vi "Auto Gyro.vi"(8 "zeroGyro":dbl, 9 "headingTarget":dbl, 10 "xSpeed":dbl) -> (1 "Finished?":bool)   [LabVIEW 2016]
uses:
  Robot Global Data.vi
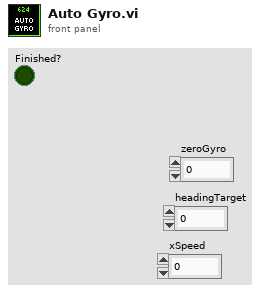
[diagram p1: front panel]
types:
  T1 = typedef "Dashboard Display Data.ctl" = cluster{"Climb Status Cluster":T2, "Drivetrain Status Cluster":T3, "Intake Status Cluster":T4, "Shooter Status Cluster":T8, "Drivetrain Encoder Values":T13, "Auton Command Cluster":T15, "Auton File Lists":T16}
  T2 = typedef "Climb Status Cluster.ctl" = cluster{"Climb Speed":dbl}
  T3 = typedef "Drivetrain Status Cluster.ctl" = cluster{"Drivetrain Mode":enum16{"Manual", "Gyro Steer"}, "Y (Throttle)":dbl, "X (Steer)":dbl, "Z (Strafe)":dbl, "Heading Target":dbl, "Center Piston Down?":bool, "Traction?":bool, "Gyro Steer Finished?":bool, "Distance Drive Finished?":bool, "Gyro":dbl, "Distance Target":dbl, "Y Max Output":dbl, "Y Min Output":dbl, "X Max Output":dbl, "X Min Output":dbl, "Z Max Output":dbl, "Z Min Output":dbl, "Translation Target":dbl, "Translation Drive Finished?":bool, "PID Auto Drive Finished?":bool, "Brake?":bool, "Vision Aligned?":bool}
  T4 = typedef "Intake Status Cluster.ctl" = cluster{"Roller Power":dbl, "Intake Mode":T5, "Intake Auto State":T6, "Backward Tripped?":bool, "Forward Tripped?":bool, "Filling Hopper?":bool, "Intake Current Trip State":T7, "Getting Gear?":bool, "Gear Slot Open":bool, "Wings Open":bool}
  T5 = typedef "Intake Modes.ctl" = enum16{"Manual", "Auto"}
  T6 = typedef "Intake Auto States.ctl" = enum16{"Outake Ball", "Idle", "Load Ball"}
  T7 = typedef "Intake Trip States.ctl" = enum16{"Normal", "Backward Tripped", "Forward Tripped"}
  T8 = typedef "Shooter Status Cluster.ctl" = cluster{"RPM":dbl, "Shooter RPM Ready?":bool, "Hopper Speed":dbl, "Shooter Mode":T9, "Shot Type":T10, "Shooter State":T11, "Motor Operational Status":T12}
  T9 = typedef "Shooter Modes.ctl" = enum16{"Auto", "Manual"}
  T10 = typedef "Shot Type.ctl" = enum16{"Dist Shot", "Key Shot"}
  T11 = typedef "Shooter Commands.ctl" = enum16{"Idle ", "Warmup ", "Shoot"}
  T12 = typedef "Shooter Motor Operational Status .ctl" = cluster{"Sensor Velocity ":dbl, "Encoder Position":dbl, "Encoder Velocity ":dbl, "Encoder Index Count":dbl, "Analog In":dbl, "Analog In Velocity":dbl, "Temperature (C)":dbl, "Temperature (K)":dbl, "Battery Voltage":dbl, "Current":dbl, "Sensor Position":dbl, "Vel Div 4":bool, "Encoder A Pin State":bool, "Encoder B Pin State":bool, "Encoder Index Pin State":bool, "Pulse Width Velocity ":dbl}
  T13 = typedef "Drivetrain Encoder Values.ctl" = cluster{"Left Encoder":T14, "Center Encoder":T14, "Right Encoder":T14}
  T14 = typedef "Encoder Values.ctl" = cluster{"Distance":dbl, "Speed":dbl, "Tick":dbl}
  T15 = typedef "Auton Command Cluster.ctl" = cluster{"commandID":dbl, "maxTime":dbl, "distanceTarget":dbl, "headingTarget":dbl, "translationTarget":dbl, "ySpeed":dbl, "xSpeed":dbl, "zSpeed":dbl, "async":dbl, "RPM":dbl, "Hood?":dbl, "Hopper?":dbl, "rollerPower":dbl, "fillHopper?":dbl, "zeroGyro":dbl}
  T16 = typedef "Auton File Lists.ctl" = cluster{"Current Queue":string, "General Scripts":string, "Movements":string}
  T17 = typedef "Drivetrain Command Cluster.ctl" = cluster{"Drivetrain Mode":T18, "Heading Target":dbl, "Turn Power":dbl, "Y Power":dbl, "Center Piston Down?":bool, "Traction?":bool, "Strafe Power":dbl, "Zero Gyro":bool, "Distance Target":dbl, "Strafe Correct":bool, "Y Max Output":dbl, "Y Min Output":dbl, "X Max Output":dbl, "X Min Output":dbl, "Z Max Output":dbl, "Z Min Output":dbl, "Z Target":dbl, "Brake?":bool}
  T18 = typedef "Drivetrain Mode.ctl" = enum16{"Manual", "Gyro Steer", "Distance Drive", "Translate Drive", "Goal Vision Align", "PID Drive"}
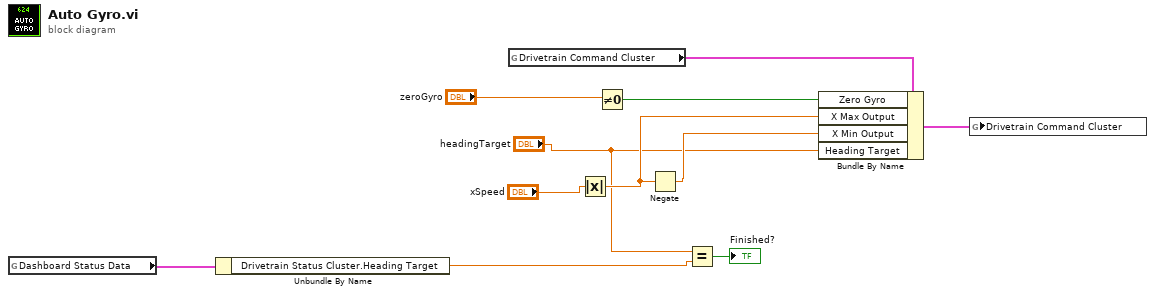
[diagram p0: block diagram]
diagram:
  n1 = global read "Robot Global Data.vi" "Dashboard Status Data"() -> (w9:T1)
  n2 = Unbundle By Name(w9) -> ("Drivetrain Status Cluster.Heading Target"=w3:dbl)
  n3 = global read "Robot Global Data.vi" "Drivetrain Command Cluster"() -> (w11:T17)
  n4 = Absolute Value(x="xSpeed") -> (abs(x)=w4:dbl)
  n5 = Not Equal To 0?(x="zeroGyro") -> (x != 0?=w8:bool)
  n6 = Negate(x=w4) -> (-x=w5:dbl)
  n7 = Equal?(x="headingTarget", y=w3) -> (x = y?=→"Finished?":bool)
  n8 = Bundle By Name(cluster=w11, "Zero Gyro"=w8, "X Max Output"=w4, "X Min Output"=w5, "Heading Target"="headingTarget") -> (w10:T17)
  n9 = global write "Robot Global Data.vi" "Drivetrain Command Cluster"(w10) -> ()
